vi "cRIO FPGA Personality.vi"() -> ()   [LabVIEW 2019]
uses:
  <vilib>/rvi/Emulation/niFpgaGetClockAttributes.vi
  <vilib>/rvi/Emulation/niFpgaSctlEmulationGetInTimedLoop.vi
  <vilib>/rvi/Emulation/niFpgaEmulationReportErrorSimple.vi
  <vilib>/rvi/Emulation/niFpgaCriticalErrorInLSC.vi
panel:
  out "Element":sgl
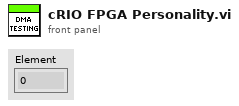
[diagram p1: front panel]
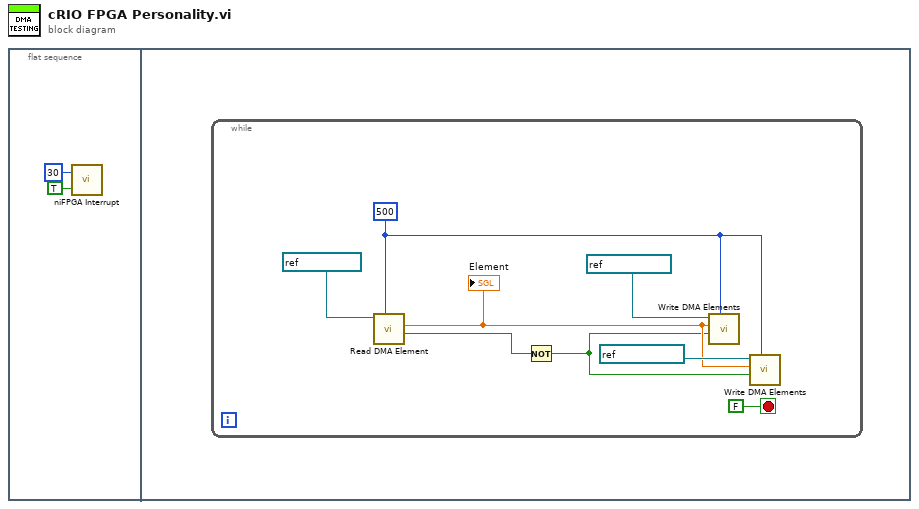
[diagram p0: block diagram]
diagram:
  n1 = flat-sequence {
    frame #0 {
      n2 = call <vilib>:"niFPGA Interrupt.vi"("Wait Until Cleared (F)"=TRUE, "IRQ Number (0)"=u8 30) -> ()  [unwired: 1 in]
    }
    frame #1 {
      n3 = while {
        stop <- FALSE stop-if-true
        w4 = 500 ("Timeout")
        n4 = call "Read DMA Element.vi"("Timeout"=w4, "DMA Refnum in"=refnum<k21> "Incoming" ("FIFO In")) -> ("isTimeout ?"=w7:bool, "DMA Element"=w5:sgl)  [unwired: 7 in, 1 out]
        "Element" <- w5
        n5 = Not(x=w7) -> (.not. x?=w3:bool)
        n6 = call "Write DMA Elements.vi"("Timeout"=w4, "isValid ?"=w3, "DMA Element"=w5, "FIFO Refnum in"=refnum<k21> "Outgoing1" ("FIFO In")) -> ()  [unwired: 7 in, 1 out]
        n7 = call "Write DMA Elements.vi"("Timeout"=w4, "isValid ?"=w3, "DMA Element"=w5, "FIFO Refnum in"=refnum<k21> "Outgoing2" ("FIFO In")) -> ()  [unwired: 7 in, 1 out]
      }
    }
  }
